vi "set encoder pos.vi"(8 "error in (no error)":errorcluster, 10 "value":i32, 11 "ch":i32) -> (0 "error out":errorcluster, 3 "function return":i32)   [LabVIEW 2014, in "test_IMU.lvlib"]
doc: "int set_encoder_pos(int ch, int value);"
uses:
  <userlib>/test_IMU/test_IMU.lvlib
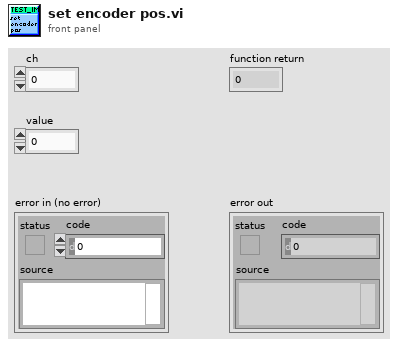
[diagram p1: front panel]
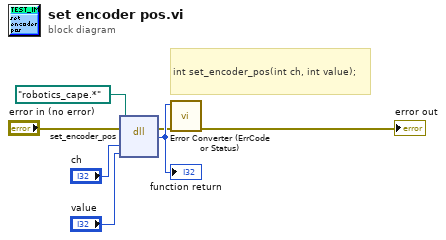
[diagram p0: block diagram]
diagram:
  # "int set_encoder_pos(int ch, int value);"
  n1 = dll-call lib="C:/Users/ktalke/Documents/Updated Header File/6.18.16/Compiled SO -schroot/robotics_cape.so" fn="set_encoder_pos"(path in=path "robotics_cape.*", error in="error in (no error)", "ch"="ch", "value"="value") -> (error out=w3:errorcluster, "return type"=w7:i32)  [unwired: 3 in, 1 out]
  "function return" <- w7
  n2 = call <userlib>:"Error Converter (ErrCode or Status).vi"("error in (no error)"=w3, "error code"=w7) -> ("error out"=→"error out":errorcluster)  [unwired: 9 in]
